vi "stringArray2String.vi"(1 "字符串数组":string[](array[string])) -> (0 "字符串":string)   [LabVIEW 2018]
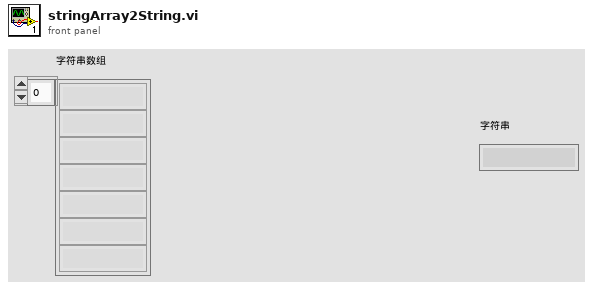
[diagram p1: front panel]
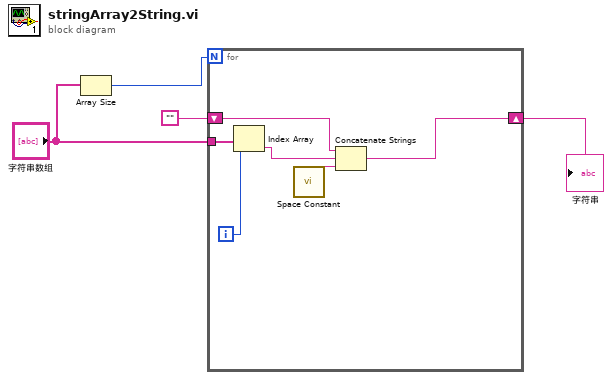
[diagram p0: block diagram]
diagram:
  n1 = Array Size(array="字符串数组") -> (size(s)=w4:i32)
  n2 = for {
    N: w4 -> [_]
    shift-right: [w10] -> w1
    shift-left: "" -> [w6]
    tunnel: "字符串数组" -> [w9]
    i -> [w8]
    n3 = Index Array(array=w9, index=w8) -> (element=w7:string)
    n4 = call <vilib>:"Space Constant.vi"() -> ("String"=w5:string)
    n5 = Concatenate Strings(w6, w7, w5) -> (w10:string)
  }
  "字符串" <- w1
